vi "LED_Globals.vi"() -> ()   [LabVIEW 2018]
panel:
  out "Visited_Disabled":bool
  out "Hatch_Ready":bool
  out "Score_Mode":bool
  out "Climbing":bool
  in  "LED_Canifier":string="LED_Canifier"
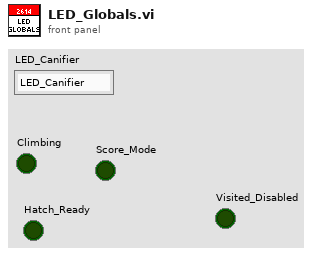
[diagram p1: front panel]
diagram:
